vi "OpenDB.vi"(8 "error in (no error)":errorcluster, 11 "DB File Name":string="temp") -> (0 "error out":errorcluster, 3 "SQLite Connection out":refnum<class "Connection.lvclass">)   [LabVIEW 2015, in "DBToolkit.lvlib"]
uses:
  DBToolkit.lvlib
  <vilib>/drjdpowell/SQLite Library/SQL Connection/Connection.lvclass
  <vilib>/drjdpowell/SQLite Library/SQL Connection/Open (path).vi
  <vilib>/drjdpowell/SQLite Library/SQL Connection/Open (string).vi
  <vilib>/AdvancedString/Path To Command Line String.vi
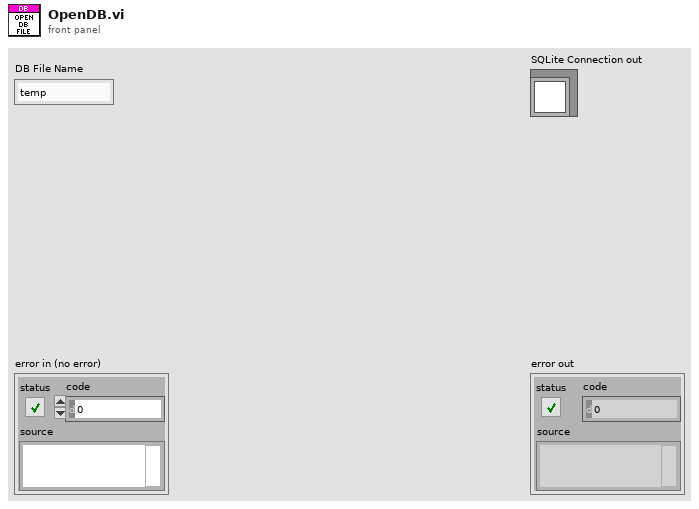
[diagram p1: front panel]
types:
  T1 = enum16{"New or existing", "Existing", "Read only"}
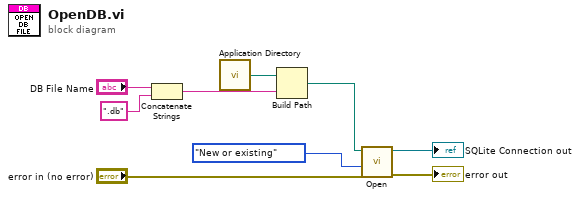
[diagram p0: block diagram]
diagram:
  n1 = Concatenate Strings("DB File Name", ".db" ("string")) -> (w3:string)
  n2 = call <vilib>:"Application Directory.vi"() -> ("Application Directory"=w8:path)
  n3 = Build Path(base path=w8, name or relative path=w3) -> (appended path=w7:path)
  n4 = call-poly <vilib>:"Open.vi"("error in (no error)"="error in (no error)", "File Option"=T1."New or existing", "db file"=w7) -> ("error out"=→"error out":errorcluster, "SQLite Connection out"=→"SQLite Connection out":refnum<class "Connection.lvclass">)  [unwired: 7 in]
